vi "Wait for Cycle.vi"(8 "error in":errorcluster, 11 "HL Timer in":refnum<class "Loop Timer.lvclass">) -> (0 "error out":errorcluster, 1 "Cycle Count":dbl, 2 "Relative Time (s)":dbl, 3 "HL Timer out":refnum<class "Loop Timer.lvclass">)   [LabVIEW 2020, in "hse-misc.lvlib" / "Loop Timer.lvclass"]
doc: "Waits until the next time cycle is reached.\n\n____\nHAMPEL SOFTWARE ENGINEERING v3.8.0 (2023-12-18 14:41)"
uses:
  Loop Timer.lvclass
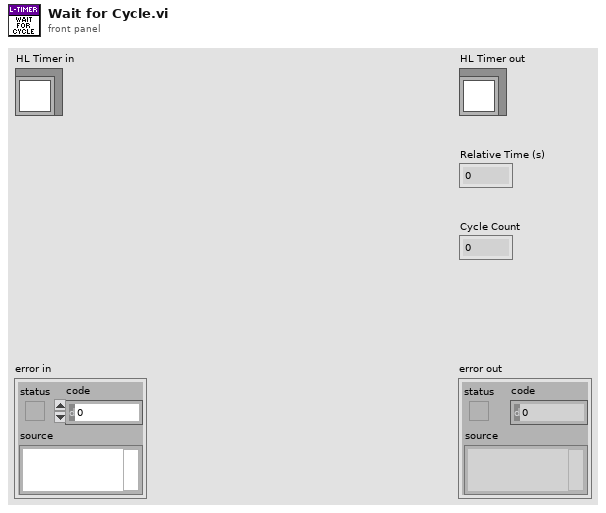
[diagram p1: front panel]
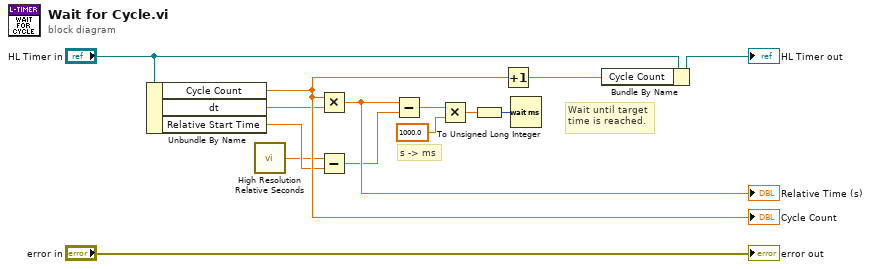
[diagram p0: block diagram]
diagram:
  # "Wait until target\ntime is reached."
  # "s -> ms"
  n1 = Unbundle By Name("HL Timer in") -> ("Cycle Count"=w9:dbl, "dt"=w8:dbl, "Relative Start Time"=w7:dbl)
  "Cycle Count" <- w9
  n2 = call <vilib>:"High Resolution Relative Seconds.vi"() -> ("relative seconds"=w6:dbl)
  n3 = Multiply(x=w9, y=w8) -> (x*y=w11:dbl)
  "Relative Time (s)" <- w11
  n4 = Subtract(x=w6, y=w7) -> (x-y=w5:dbl)
  n5 = Subtract(x=w11, y=w5) -> (x-y=w4:dbl)
  n6 = Multiply(x=w4, y=1000.0) -> (x*y=w1:dbl)
  n7 = To Unsigned Long Integer(number=w1) -> (unsigned 32bit integer=w2:u32)
  n8 = Increment(x=w9) -> (x+1=w10:dbl)
  n9 = Wait (ms)(milliseconds to wait=w2) -> ()  [unwired: 1 out]
  n10 = Bundle By Name(cluster="HL Timer in", "Cycle Count"=w10) -> (→"HL Timer out":refnum<class "Loop Timer.lvclass">)
  "error out" <- "error in"
